vi "Pockels-Generate ref frame AO sequence.vi"(6 "Cluster":T1, 8 "Previous excess us (us)":dbl, 11 "Imaging Protocol":T3) -> (0 "Excess (us)":dbl, 1 "Output sequence length (ms) (corrected for input excess)":dbl format="%#_g ms", 2 "Theoretical acquisition duration of ref frame (us)":dbl, 3 "Pockels modulation sequence":dbl[](array[numeric]), 4 "Points in o/p sequence":i32 format="%.0f points")   [LabVIEW 2020]
uses:
  Typedefs/Imaging Protocols enum.ctl
  Typedefs/Pockels modulation Internal cluster 1.ctl
  Typedefs/Rounding type.ctl
  Typedefs/Pockels mod gen variables cluster.ctl
  Globals/gl_Pockels control globals.vi
  Global Variables/General Globals.vi
  User Interface/Movement Correction/Globals/gl_Movement correction globals.vi
panel:
  out "Multi-line pockels modulation waveform":dbl[](graph)
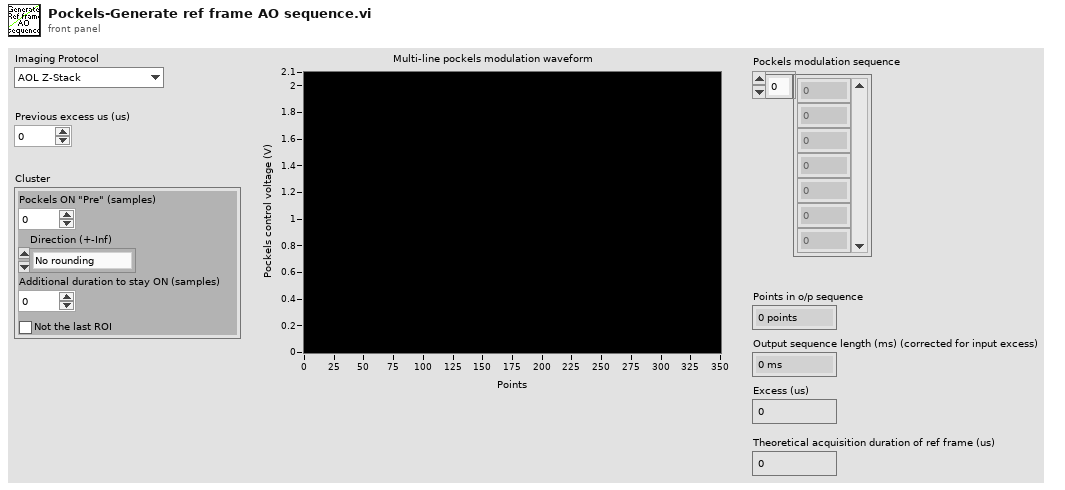
[diagram p1: front panel]
types:
  T1 = typedef "Pockels modulation Internal cluster 1.ctl" = cluster{"Pockels ON \"Pre\" (samples)":i32, "Direction (+-Inf)":T2, "Additional duration to stay ON (samples)":i32, "Not the last ROI":bool}
  T2 = typedef "Rounding type.ctl" = enum16{"No rounding", "Toward +Inf", "Toward -Inf"}
  T3 = typedef "Imaging Protocols enum.ctl" = enum16{"AOL Z-Stack", "Motor Z Stack", "Functional Acquisition", "Single Plane Acquisition", "Volume Acquisition", "Live Imaging", "Live Plane Imaging", "Live Volume Imaging"}
  T4 = typedef "Pockels mod gen variables cluster.ctl" = cluster{"Dwell time":dbl, "Number of frame lines":i32, "Number of points in a line":i32, "Index of Z-plane":i32, "Pockels \"Low\" time (us)":dbl, "Sample Clock Rate":dbl, "Imaging Protocol":T3}
  T5 = typedef "Ref DAQ Param.ctl" = cluster{"Full Frame Size":u16, "Ref Field of View":sgl, "Ref Zoom":i8, "Ref_dwellTime":sgl, "Ref X-pixels-per-line(Npxr)":i16, "Ref Y-lines-per-image(Npyr)":i16, "Ref Z-lines-per-image":i16, "Ignore Z lines":i16, "Ref Scan Cycles":i32, "Ref threshold XY":u16, "Ref threshold Z":u16, "Ref average XY":u16, "Ref Average  Z":u16, "Proportional_scale":fxp<+,16,2>, "Integral_scale":fxp<+/-,16,12>, "Proportional_scale Z":fxp<+,16,2>, "Integral_scale Z":fxp<+/-,16,12>, "Diff_threshold":fxp<+,16,2>, "Diff_threshold _z":fxp<+,16,2>, "Sliding Average":bool, "Ref count reset enabled":bool}
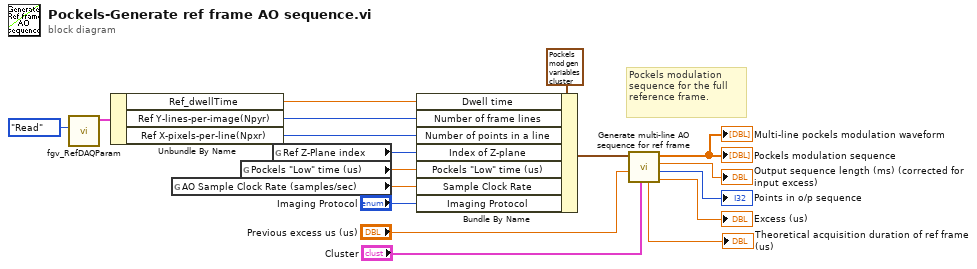
[diagram p0: block diagram]
diagram:
  # "Pockels modulation sequence for the full reference frame."
  n1 = call "fgv_RefDAQParam.vi"("Function"=enum16{"Initialize", "Write", "Read"}."Read" ("Status")) -> ("RefDAQParam"=w10:T5)  [unwired: 9 in, 1 out]
  n2 = Unbundle By Name(w10) -> ("Ref_dwellTime"=w14:sgl, "Ref Y-lines-per-image(Npyr)"=w12:i16, "Ref X-pixels-per-line(Npxr)"=w13:i16)
  n3 = global read "General Globals.vi" "AO Sample Clock Rate (samples/sec)"() -> (w18:dbl)
  n4 = global read "gl_Pockels control globals.vi" "Pockels \"Low\" time (us)"() -> (w17:dbl)
  n5 = global read "gl_Movement correction globals.vi" "Ref Z-Plane index"() -> (w9:i32)
  n6 = Bundle By Name(cluster=T4 {"Dwell time"=0.0, "Number of frame lines"=512, "Number of points in a line"=0, "Index of Z-plane"=0, "Pockels \"Low\" time (us)"=0.0, "Sample Clock Rate"=0.0, "Imaging Protocol"=enum."AOL Z-Stack"} ("Variables"), "Dwell time"=w14, "Number of frame lines"=w12, "Number of points in a line"=w13, "Index of Z-plane"=w9, "Pockels \"Low\" time (us)"=w17, "Sample Clock Rate"=w18, "Imaging Protocol"="Imaging Protocol") -> (w8:T4)
  n7 = call "Generate multi-line AO sequence for ref frame.vi"("Cluster"="Cluster", "Previous excess us (us)"="Previous excess us (us)", "Variables"=w8) -> ("Excess (us)"=→"Excess (us)":dbl, "Points in o/p sequence"=→"Points in o/p sequence":i32, "Output sequence length (ms)"=→"Output sequence length (ms) (corrected for input excess)":dbl, "Pockels modulation sequence"=→"Pockels modulation sequence" →"Multi-line pockels modulation waveform":dbl[], "Theoretical acquisition duration of ref frame (us)"=→"Theoretical acquisition duration of ref frame (us)":dbl)  [unwired: 4 in]
